vi "Create UEs.vi"(11 "ABD Panel in":refnum<class "ABD Panel.lvclass">) -> (0 "error out":errorcluster, 3 "ABD Panel out":refnum<class "ABD Panel.lvclass">)   [LabVIEW 2021, in "ABD Panel.lvclass"]
uses:
  ABD Panel.lvclass
  ABD Panel.lvclass/ABD Panel.ctl
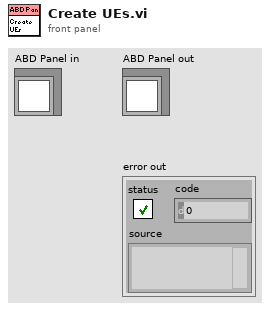
[diagram p1: front panel]
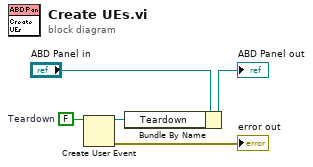
[diagram p0: block diagram]
diagram:
  w5 = FALSE  # Teardown
  n1 = Create User Event(user event datatype=w5) -> (user event=w1:refnum<user-event>, error out=→"error out":errorcluster)  [unwired: 1 in]
  n2 = Bundle By Name(cluster="ABD Panel in", "Teardown"=w1) -> (→"ABD Panel out":refnum<class "ABD Panel.lvclass">)
